vi "LCS assignemnts.vi"(9 "cluster centers":string[](array[string])=["1 0 -1 1 -1 0 -4 1 -4 0 1", "2 0 -1 2 -1 0 -2 2 -2 0 2", "3 0 -3 3 -3 0 -2 3 -2 0 3", "4 0 -3 4 -3 0 -4 4 -4 0 4", "-1 1 -4 0 -4 4 -3 4 -4 0 -4 1 -1", "-1 2 -2 0 -2 3 -3 3 -2 0 -2 2 -1", "-4 1 -1 0 -1 2 -2 2 -1 0 -1 1 -4", "-4 4 -3 0 -3 3 -2 3 -3 0 -3 4 -4", "0 -4 1 -1 0 -3 3 -2 3 -3 0 -1 1 -4 0", "0 -4 4 -3 0 -1 2 -2 2 -1 0 -3 4 -4 0"], 11 "Patterns in":string[](array[string])=["0 4 0", "4 0 4", "0 4 0", "4 0 4", "0 4 0", "4 0 4", "0 4 0", "4 0 -2", "0 -2 3", "-2 3 0", "3 0 3", "0 3 0", "3 0 4", "0 4 0", "-2 0 1", "0 1 0", "1 0 -4", "0 -4 4", "-2 2 0", "2 0 -1", "0 -1 -4", "-1 -4 1", "-4 1 0", "1 0 3", "0 3 0", "-1 0 -1", "0 -1 2", "0 -1 1", "-1 1 0", "1 0 4", "0 4 0", "4 0 3", "0 3 -2", "3 -2 0", "-2 0 -2", "0 -2 3", "-2 3 -2", "3 -2 0", "-2 0 4", "0 4 0", "4 0 -2", "0 -2 2", "2 -1 0", "-1 0 4", "0 4 0", "4 0 2", "0 2 0", "2 0 -2", "0 -2 0", "1 -1 0", "-1 0 3", "0 3 0", "3 0 -4", "0 -4 4", "-4 4 -4", "4 -4 0", "2 -1 0", "-1 0 3", "0 3 -2", "3 -2 0", "-2 0 -3", "0 -3 0", "-3 0 3", "0 3 0", "3 0 -3", "0 -3 0", "0 4 0", "4 0 4", "0 4 -4", "4 -4 1", "-4 1 -1", "1 -1 0", "-1 0 -3", "0 -3 0", "-3 0 1", "0 1 -4", "1 -4 1", "-4 1 0", "1 0 4", "0 4 0", "4 0 -4", "0 -4 0", "-4 0 -4", "0 -4 4", "-4 4 -4", "4 -4 1", "0 -4 1", "-4 1 0", "1 0 -4", "0 -4 4", "0 4 0", "4 0 -2", "0 -2 2", "-2 2 -2", "2 -2 2", "-2 2 -2", "2 -2 2", "-2 2 -1", "2 -1 0", "-1 0 4", "0 4 0", "4 0 2", "0 2 0", "2 0 4", "0 4 0", "4 0 2", "0 2 -2", "2 -2 0", "-2 0 4", "1 0 -1", "0 -1 0", "-1 0 -1", "0 -1 0", "-1 0 1", "0 1 -1", "-2 2 -2", "2 -2 3", "1 0 -1", "0 -1 0", "-1 0 -1", "0 -1 2", "-1 2 0", "2 0 2", "0 2 -2", "2 -2 0", "-2 0 -4", "0 -4 0", "-2 2 0", "2 0 3", "0 3 -2", "3 -2 2", "1 -1 0", "-1 0 3", "0 4 0", "-2 0 1", "0 1 -4", "1 -4 0", "-4 0 -3", "0 -3 0", "1 0 -1", "0 -1 2", "-1 2 -1", "2 -1 1", "-1 1 -4", "-2 0 -1", "0 -1 1", "0 3 0", "3 0 3", "0 3 0", "3 0 3", "0 3 -2", "-4 0 -4", "0 -4 4", "0 4 0", "4 0 -4", "0 -4 0", "-4 0 -4", "-2 2 0", "2 0 4", "0 4 -4", "4 -4 0", "-4 0 2", "0 2 -2"]) -> (0 "LCS/Lsample (zeroed)/Lknown":dbl[][](array[numeric]), 1 "Assignment (enhanced)":string[](array[string]), 2 "LCS/Lsample/Lknown":dbl[][](array[numeric]), 3 "Assigned LCS":string[](array[string]), 4 "Distance values (LCS)":dbl[][](array[numeric]), 5 "LCS/min (Lsample,Lknown)":dbl[][](array[numeric]), 6 "LCS/LA+LB-LCS":dbl[][](array[numeric]), 7 "LCS/MAX (Lsample,Lknown)":dbl[][](array[numeric]), 8 "LCS/Lrep":dbl[][](array[numeric]))   [LabVIEW 2014]
panel:
  out "LCS if = length":dbl[][](array[numeric])
  out "LCS/Lsample":dbl[][](array[numeric])
  out "L cluster centers":i32[](array[numeric])
  out "L sample":i32[](array[numeric])
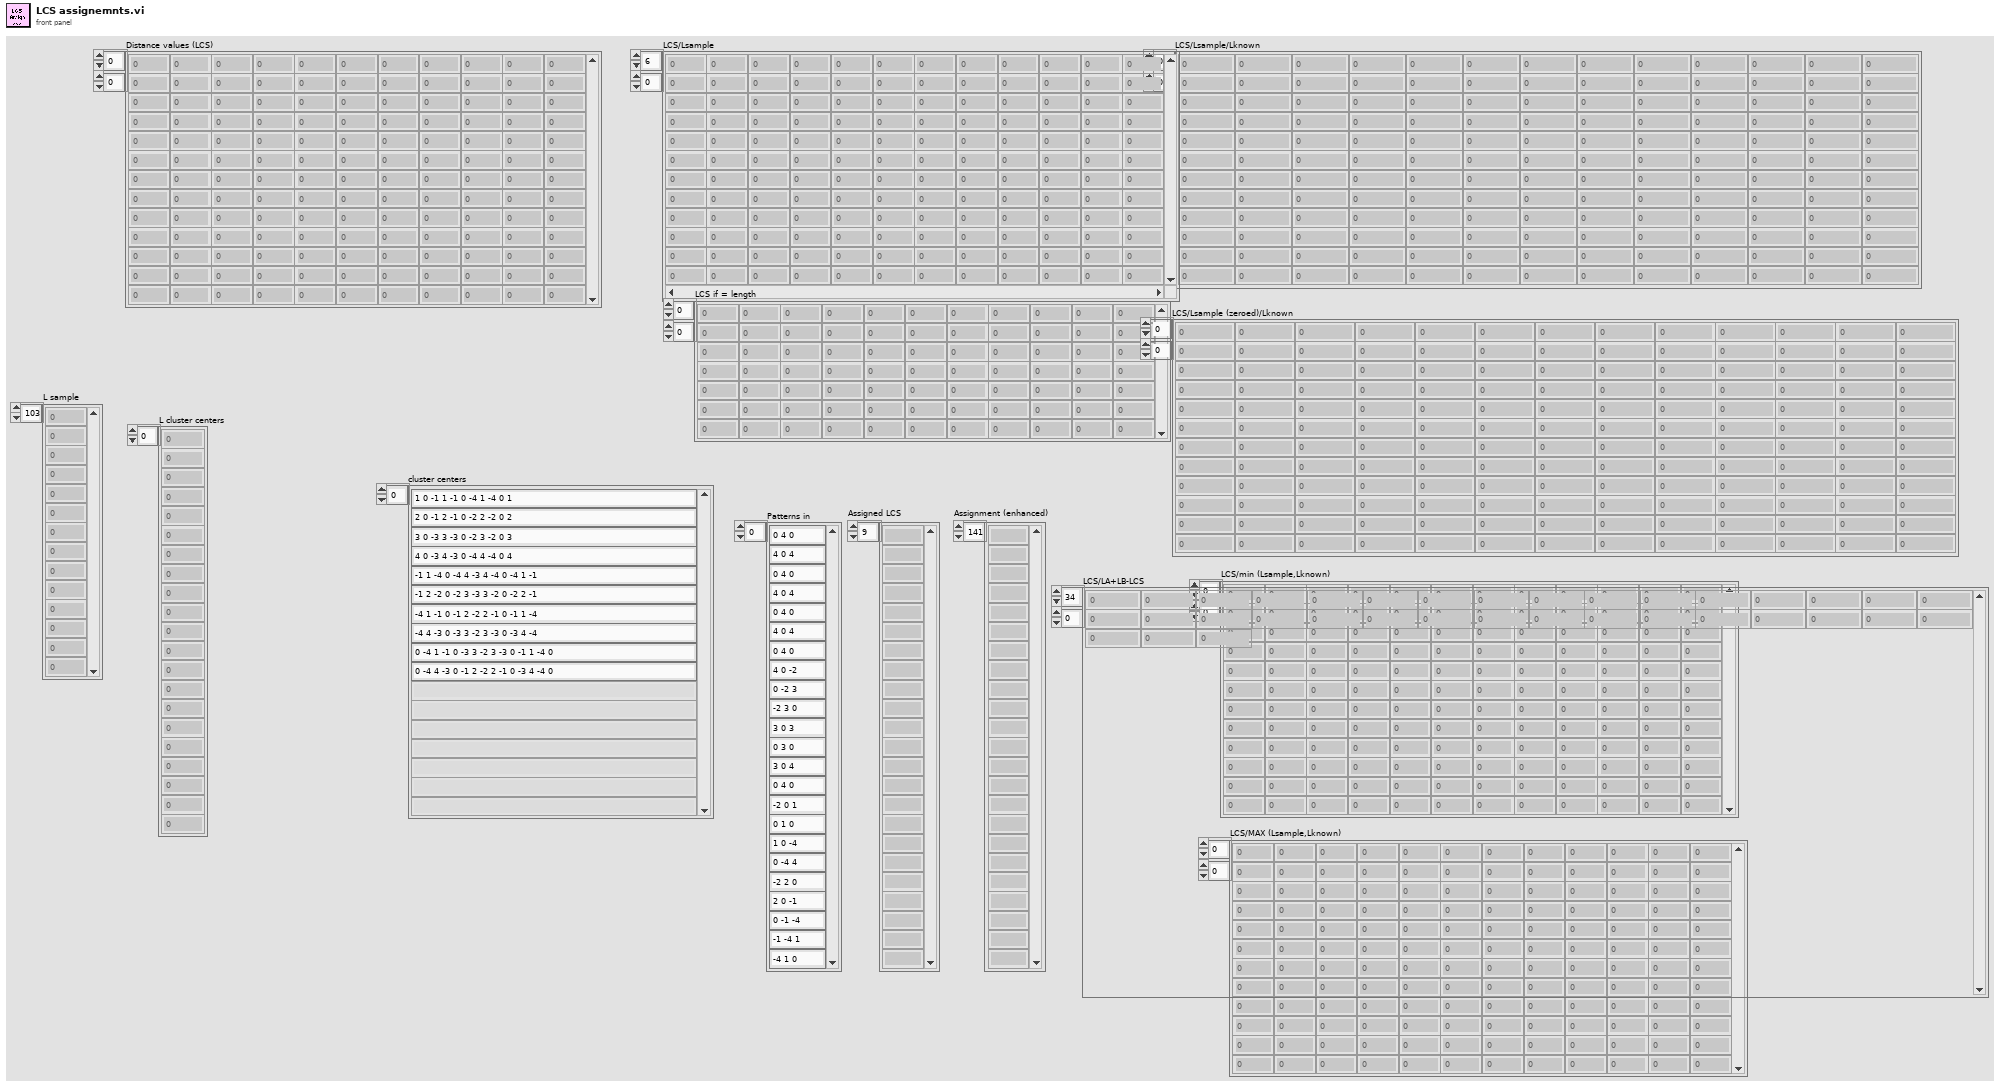
[diagram p1: front panel]
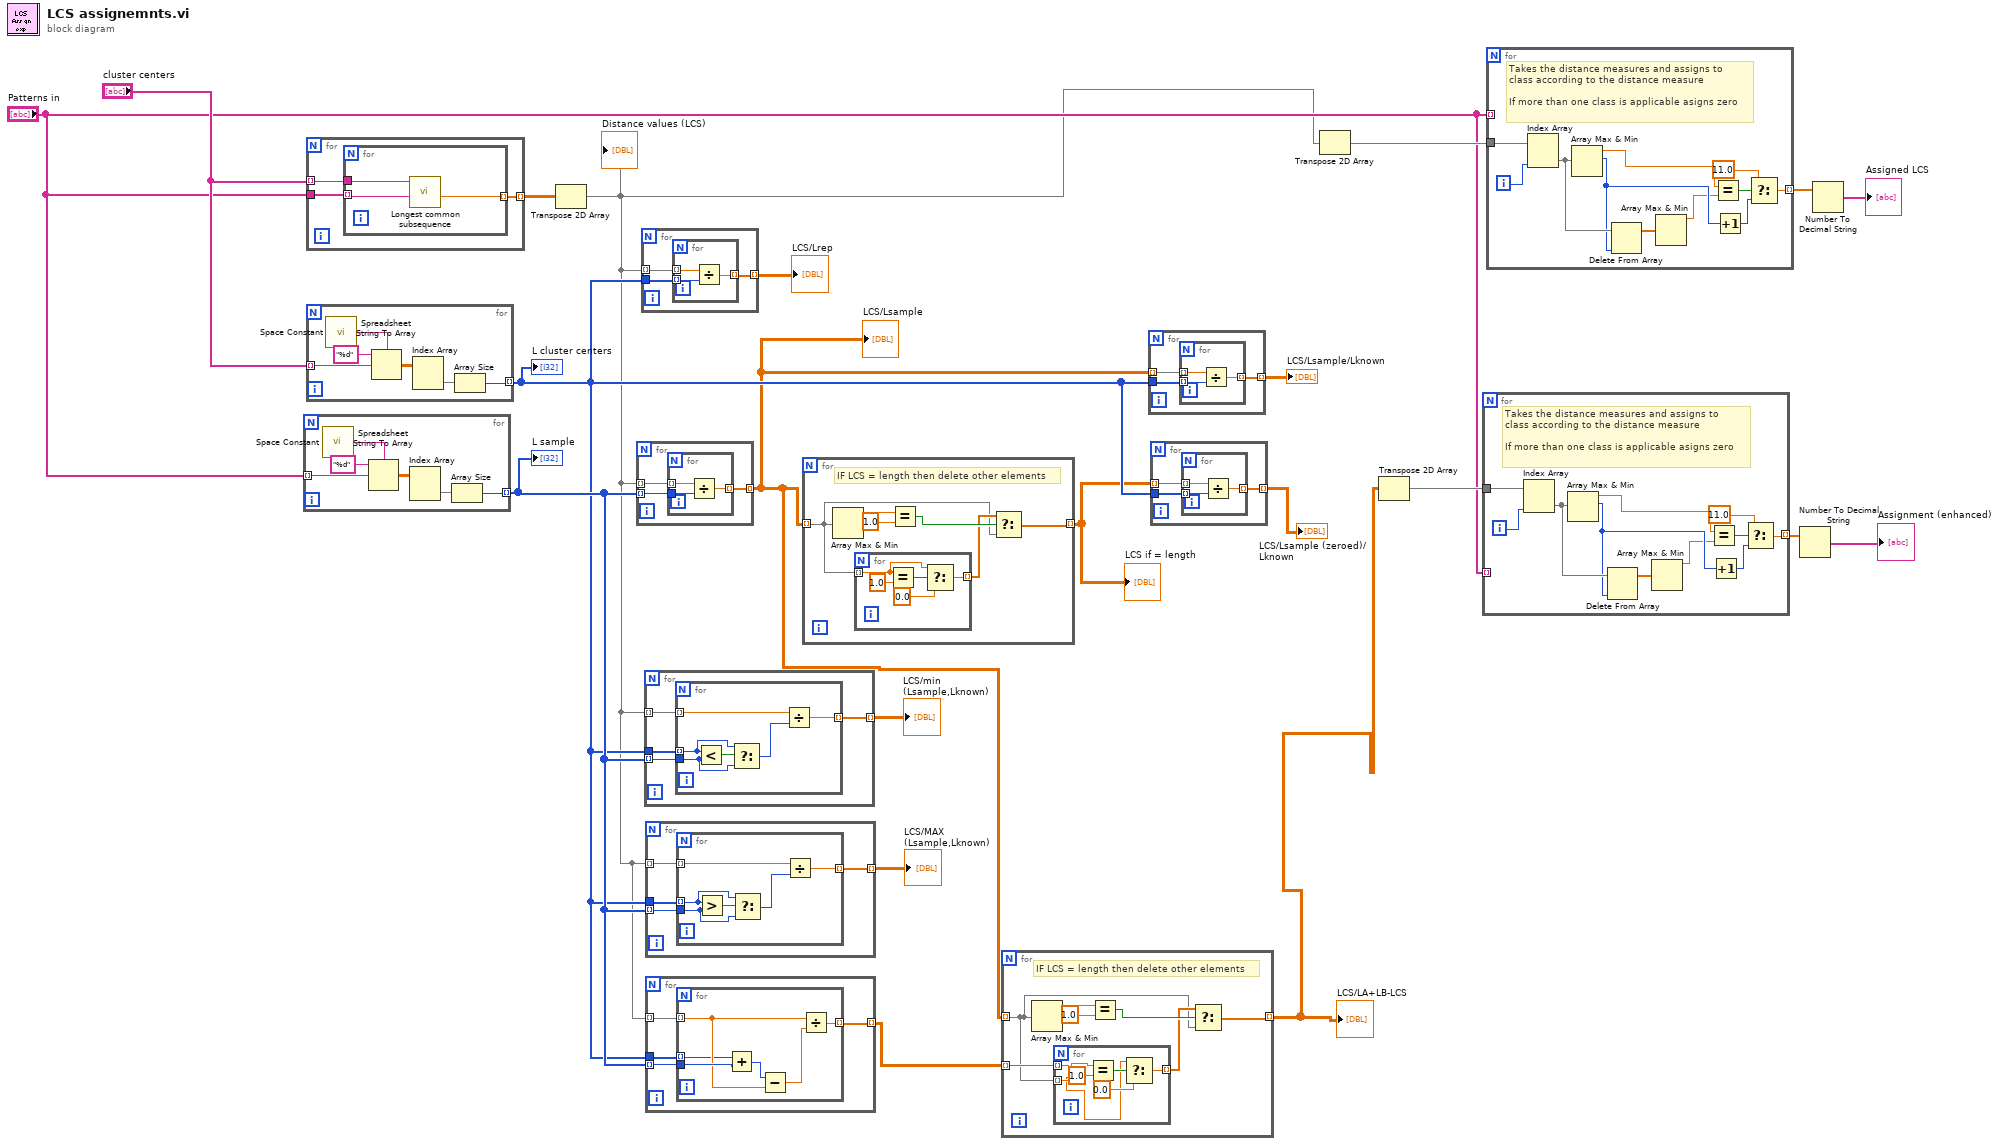
[diagram p0: block diagram]
diagram:
  n1 = for {
    tunnel: "Patterns in" -> [w26] mode=indexing
    tunnel: [w22] -> w12 mode=indexing
    n2 = call <vilib>:"Space Constant.vi"() -> ("String"=w27:string)
    n3 = Spreadsheet String To Array(delimiter (Tab)=w27, format string="%d", spreadsheet string=w26) -> (array=w24:dbl[][])  [unwired: 1 in]
    n4 = Index Array(array=w24) -> (element=w23:dbl[])  [unwired: 2 in]
    n5 = Array Size(array=w23) -> (size(s)=w22:i32)
  }
  "L sample" <- w12
  n6 = for {
    tunnel: "cluster centers" -> [w30] mode=indexing
    tunnel: [w29] -> w20 mode=indexing
    tunnel: "Patterns in" -> [w28]
    n7 = for {
      tunnel: w28 -> [w32] mode=indexing
      tunnel: w30 -> [w33]
      tunnel: [w31] -> w29 mode=indexing
      n8 = call "Longest common subsequence.vi"("Pattern 2 COLUMN(0)"=w32, "Pattern 1 ROW(0)"=w33) -> ("LCS length"=w31:dbl)  [unwired: 8 in, 1 out]
    }
  }
  n9 = for {
    tunnel: "cluster centers" -> [w38] mode=indexing
    tunnel: [w34] -> w11 mode=indexing
    n10 = call <vilib>:"Space Constant.vi"() -> ("String"=w39:string)
    n11 = Spreadsheet String To Array(delimiter (Tab)=w39, format string="%d", spreadsheet string=w38) -> (array=w36:dbl[][])  [unwired: 1 in]
    n12 = Index Array(array=w36) -> (element=w35:dbl[])  [unwired: 2 in]
    n13 = Array Size(array=w35) -> (size(s)=w34:i32)
  }
  "L cluster centers" <- w11
  n14 = Transpose 2D Array(2D array=w20) -> (transposed array=w1:dbl[][])
  "Distance values (LCS)" <- w1
  n15 = for {
    tunnel: w1 -> [w42] mode=indexing
    tunnel: w12 -> [w41] mode=indexing
    tunnel: [w40] -> w2 mode=indexing
    n16 = for {
      tunnel: w42 -> [w45] mode=indexing
      tunnel: w41 -> [w44]
      tunnel: [w43] -> w40 mode=indexing
      n17 = Divide(x=w45, y=w44) -> (x/y=w43:dbl)
    }
  }
  "LCS/Lsample" <- w2
  n18 = for {
    tunnel: w1 -> [w48] mode=indexing
    tunnel: w11 -> [w47]
    tunnel: [w46] -> w8 mode=indexing
    n19 = for {
      tunnel: w48 -> [w51] mode=indexing
      tunnel: w47 -> [w49] mode=indexing
      tunnel: [w50] -> w46 mode=indexing
      n20 = Divide(x=w51, y=w49) -> (x/y=w50:dbl)
    }
  }
  "LCS/Lrep" <- w8
  n21 = for {
    tunnel: w1 -> [w55] mode=indexing
    tunnel: w12 -> [w52] mode=indexing
    tunnel: [w54] -> w10 mode=indexing
    tunnel: w11 -> [w53]
    n22 = for {
      tunnel: w55 -> [w61] mode=indexing
      tunnel: [w60] -> w54 mode=indexing
      tunnel: w53 -> [w58] mode=indexing
      tunnel: w52 -> [w57]
      n23 = Less?(x=w58, y=w57) -> (x < y?=w59:bool)
      n24 = Select(t=w58, s=w59, f=w57) -> (s? t:f=w56:i32)
      n25 = Divide(x=w61, y=w56) -> (x/y=w60:dbl)
    }
  }
  "LCS/min (Lsample,Lknown)" <- w10
  n26 = for {
    tunnel: w1 -> [w65] mode=indexing
    tunnel: w12 -> [w62] mode=indexing
    tunnel: [w64] -> w9 mode=indexing
    tunnel: w11 -> [w63]
    n27 = for {
      tunnel: w65 -> [w71] mode=indexing
      tunnel: [w70] -> w64 mode=indexing
      tunnel: w63 -> [w68] mode=indexing
      tunnel: w62 -> [w67]
      n28 = Greater?(x=w68, y=w67) -> (0:w69:bool)
      n29 = Select(t=w68, s=w69, f=w67) -> (s? t:f=w66:i32)
      n30 = Divide(x=w71, y=w66) -> (x/y=w70:dbl)
    }
  }
  "LCS/MAX (Lsample,Lknown)" <- w9
  n31 = for {
    tunnel: w1 -> [w75] mode=indexing
    tunnel: w12 -> [w72] mode=indexing
    tunnel: [w74] -> w4 mode=indexing
    tunnel: w11 -> [w73]
    n32 = for {
      tunnel: w75 -> [w79] mode=indexing
      tunnel: [w81] -> w74 mode=indexing
      tunnel: w73 -> [w77] mode=indexing
      tunnel: w72 -> [w80]
      n33 = Add(x=w77, y=w80) -> (x+y=w76:i32)
      n34 = Subtract(x=w76, y=w79) -> (x-y=w78:dbl)
      n35 = Divide(x=w79, y=w78) -> (x/y=w81:dbl)
    }
  }
  n36 = for {
    tunnel: w2 -> [w82] mode=indexing
    tunnel: [w84] -> w7 mode=indexing
    # "IF LCS = length then delete other elements"
    n37 = Array Max & Min(array=w82) -> (max value=w87:dbl)  [unwired: 3 out]
    n38 = for {
      tunnel: w82 -> [w88] mode=indexing
      tunnel: [w89] -> w83 mode=indexing
      n39 = Equal?(x=w88, y=1.0) -> (x = y?=w92:bool)
      n40 = Select(t=w88, s=w92, f=0.0) -> (s? t:f=w89:dbl)
    }
    n41 = Equal?(x=w87, y=1.0) -> (x = y?=w85:bool)
    n42 = Select(t=w83, s=w85, f=w82) -> (s? t:f=w84:dbl[])
  }
  "LCS if = length" <- w7
  n43 = for {
    tunnel: w2 -> [w93] mode=indexing
    tunnel: [w96] -> w3 mode=indexing
    tunnel: w4 -> [w94] mode=indexing
    # "IF LCS = length then delete other elements"
    n44 = Array Max & Min(array=w93) -> (max value=w99:dbl)  [unwired: 3 out]
    n45 = for {
      tunnel: w94 -> [w100] mode=indexing
      tunnel: [w102] -> w95 mode=indexing
      tunnel: w93 -> [w101] mode=indexing
      n46 = Equal?(x=w101, y=1.0) -> (x = y?=w105:bool)
      n47 = Select(t=w100, s=w105, f=0.0) -> (s? t:f=w102:dbl)
    }
    n48 = Equal?(x=w99, y=1.0) -> (x = y?=w97:bool)
    n49 = Select(t=w95, s=w97, f=w93) -> (s? t:f=w96:dbl[])
  }
  "LCS/LA+LB-LCS" <- w3
  n50 = for {
    tunnel: w2 -> [w108] mode=indexing
    tunnel: w11 -> [w107]
    tunnel: [w106] -> w6 mode=indexing
    n51 = for {
      tunnel: w108 -> [w111] mode=indexing
      tunnel: w107 -> [w109] mode=indexing
      tunnel: [w110] -> w106 mode=indexing
      n52 = Divide(x=w111, y=w109) -> (x/y=w110:dbl)
    }
  }
  "LCS/Lsample/Lknown" <- w6
  n53 = for {
    tunnel: w7 -> [w114] mode=indexing
    tunnel: w11 -> [w113]
    tunnel: [w112] -> w5 mode=indexing
    n54 = for {
      tunnel: w114 -> [w117] mode=indexing
      tunnel: w113 -> [w115] mode=indexing
      tunnel: [w116] -> w112 mode=indexing
      n55 = Divide(x=w117, y=w115) -> (x/y=w116:dbl)
    }
  }
  "LCS/Lsample (zeroed)/Lknown" <- w5
  n56 = Transpose 2D Array(2D array=w1) -> (transposed array=w21:dbl[][])
  n57 = Transpose 2D Array(2D array=w3) -> (transposed array=w16:dbl[][])
  n58 = for {
    tunnel: w16 -> [w128]
    tunnel: [w118] -> w17 mode=indexing
    tunnel: "Patterns in" -> [_] mode=indexing
    i -> [w127]
    # "Takes the distance measures and assigns to \nclass according to the distance measure\n\nIf more than one class is applicable asigns zero"
    n59 = Index Array(array=w128, index (col)=w127) -> (element=w122:dbl[])  [unwired: 1 in]
    n60 = Array Max & Min(array=w122) -> (max value=w121:dbl, max index (indices)=w120:i32)  [unwired: 2 out]
    n61 = Delete From Array(array=w122, index=w120) -> (array with subset deleted=w126:dbl[])  [unwired: 1 in, 1 out]
    n62 = Array Max & Min(array=w126) -> (max value=w119:dbl)  [unwired: 3 out]
    n63 = Equal?(x=w121, y=w119) -> (x = y?=w125:bool)
    n64 = Increment(x=w120) -> (x+1=w123:i32)
    n65 = Select(t=11.0, s=w125, f=w123) -> (s? t:f=w118:dbl)
  }
  n66 = for {
    tunnel: "Patterns in" -> [_] mode=indexing
    tunnel: w21 -> [w139]
    tunnel: [w129] -> w19 mode=indexing
    i -> [w138]
    # "Takes the distance measures and assigns to \nclass according to the distance measure\n\nIf more than one class is applicable asigns zero"
    n67 = Index Array(array=w139, index (col)=w138) -> (element=w133:dbl[])  [unwired: 1 in]
    n68 = Array Max & Min(array=w133) -> (max value=w132:dbl, max index (indices)=w131:i32)  [unwired: 2 out]
    n69 = Delete From Array(array=w133, index=w131) -> (array with subset deleted=w137:dbl[])  [unwired: 1 in, 1 out]
    n70 = Array Max & Min(array=w137) -> (max value=w130:dbl)  [unwired: 3 out]
    n71 = Equal?(x=w132, y=w130) -> (x = y?=w136:bool)
    n72 = Increment(x=w131) -> (x+1=w134:i32)
    n73 = Select(t=11.0, s=w136, f=w134) -> (s? t:f=w129:dbl)
  }
  n74 = Number To Decimal String(number=w17) -> (decimal integer string=→"Assignment (enhanced)":string[])  [unwired: 1 in]
  n75 = Number To Decimal String(number=w19) -> (decimal integer string=→"Assigned LCS":string[])  [unwired: 1 in]
